vi "GetParam.vi"(8 "error in (no error)":errorcluster caption="entrée d'erreur (pas d'erreur)", 11 "Coverage_Error.lvclass":refnum<class "Coverage_Error.lvclass">) -> (0 "error out":errorcluster caption="sortie d'erreur", 2 "coverage_error":cluster{"sample_weight":dbl[]}, 3 "Coverage_Error.lvclass":refnum<class "Coverage_Error.lvclass">)   [LabVIEW 2020, in "Coverage_Error.lvclass"]
doc: "Get Parameters"
uses:
  Coverage_Error.lvclass
  Coverage_Error.lvclass/Coverage_Error.ctl
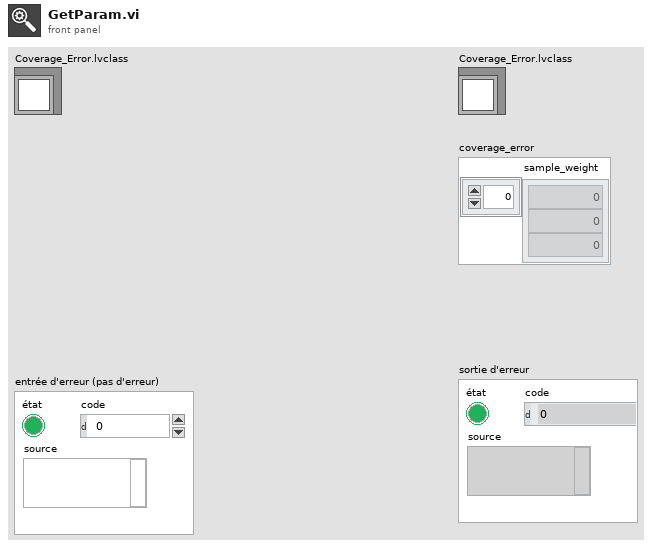
[diagram p1: front panel]
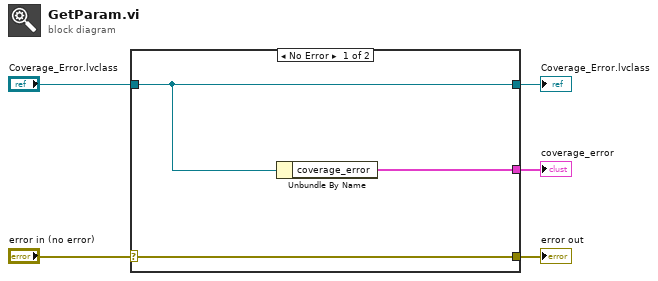
[diagram p0: block diagram]
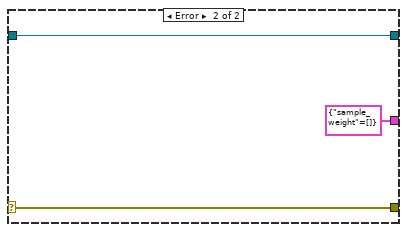
[diagram p2: hidden frame]
diagram:
  n1 = case shown="No Error" "error in (no error)" {
    selector: "error in (no error)" -> [w8 w10]
    tunnel: [w8 w10] -> w4
    tunnel: [w7 w11] -> w2
    tunnel: "Coverage_Error.lvclass" -> [w7 w11]
    tunnel: [w6 cluster{"sample_weight":dbl[]} {"sample_weight"=[]} ("coverage_error")] -> w1
    frame No Error {
      n2 = Unbundle By Name(w7) -> ("coverage_error"=w6:cluster{"sample_weight":dbl[]})
    }
    frame Error {
    }
  }
  "error out" <- w4
  "Coverage_Error.lvclass" <- w2
  "coverage_error" <- w1
